vi "Build_Script.vi"(5 "Commands":cluster{"Command":string, "Parameters":string}[](array[cluster])) -> (2 "script out":T1)   [LabVIEW 2015]
uses:
  Script.ctl
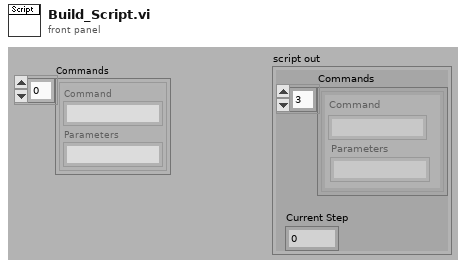
[diagram p1: front panel]
types:
  T1 = typedef "Script.ctl" = cluster{"Current Step":i32, "Commands":cluster{"Command":string, "Parameters":string}[]}
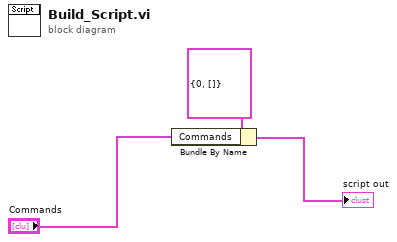
[diagram p0: block diagram]
diagram:
  n1 = Bundle By Name(cluster=T1 {"Current Step"=0, "Commands"=[]} ("Script"), "Commands"="Commands") -> (→"script out":T1)
